vi "Lookup AI.vi"(8 "error in (no error)":errorcluster, 10 "ADC #":T1=-1, 11 "Session in":refnum<class "Session.lvclass">) -> (0 "error out":errorcluster, 2 "AI":refnum<class "AI.lvclass">, 3 "Session out":refnum<class "Session.lvclass">)   [LabVIEW 2020, in "CTI.lvlib" / "Session.lvclass"]
uses:
  Session.lvclass
  ADC Number.ctl
  AI/AI.lvclass
  Session.lvclass/Session.ctl
  90ecd9bf-ac86-437b-a517-ed93800de6f7.vi
  8cbe5373-6287-4c2d-ac0f-d8c3e0aec529.vi
  90ecd9bf-ac86-437b-a517-ed93800de6f7.vi/685f7f19-b444-4620-8f66-e6e2ddd64bb8.vi
  8cbe5373-6287-4c2d-ac0f-d8c3e0aec529.vi/e2895f7d-be08-489f-ac40-10d6f32e0019.vi
  Generate Error.vi
  Resource/Resource.lvclass
  CTI.lvlib
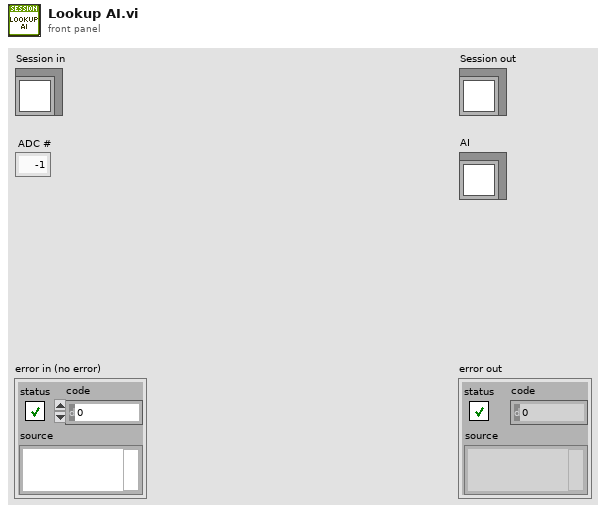
[diagram p1: front panel]
types:
  T1 = typedef "CTI.lvlib/ADC Number.ctl" = i8
  T2 = typedef "CTI.lvlib/Session.lvclass/Resources.ctl" = cluster{"GPIO":map{T3, refnum<class "GPIO.lvclass">}, "AI":map{T1, refnum<class "AI.lvclass">}, "PWM":map{T3, refnum<class "PWM.lvclass">}, "UART":map{T4, refnum<class "UART.lvclass">}, "I2C":map{T5, refnum<class "I2C.lvclass">}, "SPI":map{T6, refnum<class "SPI.lvclass">}, "CS":map{T3, refnum<class "SPI CS.lvclass">}}
  T3 = typedef "CTI.lvlib/GPIO Number.ctl" = i8
  T4 = typedef "CTI.lvlib/UART Number.ctl" = i8
  T5 = typedef "CTI.lvlib/I2C Number.ctl" = i8
  T6 = typedef "CTI.lvlib/SPI Number.ctl" = i8
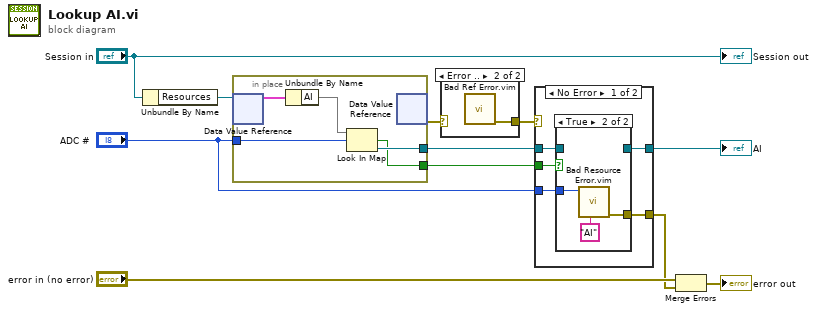
[diagram p0: block diagram]
diagram:
  n1 = Unbundle By Name("Session in") -> ("Resources"=w2:refnum<data-value>)
  n2 = in-place {
    in-place-border: "ADC #" -> [w16]
    in-place-border: [w15] -> w8
    in-place-border: [w14] -> w10
    n3 = in-place-dvr #1(w2) -> (w13:T2)  [unwired: 1 out]
    n4 = Unbundle By Name(w13) -> ("AI"=w12:map{T1, refnum<class "AI.lvclass">})
    n5 = Look In Map(map=w12, key=w16) -> (key not found?=w14:bool, value=w15:refnum<class "AI.lvclass">)  [unwired: 1 in]
    n6 = in-place-dvr #1() -> (w1:errorcluster)  [unwired: 1 in, 1 out]
  }
  n7 = case shown="Error .." w1 {
    tunnel: [_ w17] -> w9
    frame No Error {
    }
    frame Error {
      n8 = call "Bad Ref Error.vim"() -> ("error out"=w17:errorcluster)  [unwired: 10 in, 1 out]
    }
  }
  n9 = case shown="No Error" w9 {
    selector: w9 -> [_ w27]
    tunnel: w10 -> [w22 _]
    tunnel: w8 -> [w21 _]
    tunnel: [w20 _] -> w7
    tunnel: "ADC #" -> [w19 _]
    tunnel: [w18 w27] -> w3
    frame No Error {
      n10 = case shown="True" w22 {
        tunnel: w21 -> [w23 _]
        tunnel: [w23 _] -> w20
        tunnel: w19 -> [_ w26]
        tunnel: [_ w25] -> w18
        frame False {
        }
        frame True {
          n11 = call "Bad Resource Error.vim"("Resource Type"="AI", "Res #"=w26) -> ("error out"=w25:errorcluster)  [unwired: 8 in, 1 out]
        }
      }
    }
    frame Error {
    }
  }
  "AI" <- w7
  n12 = Merge Errors("error in (no error)", w3) -> (→"error out":errorcluster)
  "Session out" <- "Session in"
